vi "ArmFeedForward_Example.vi"() -> ()   [LabVIEW 2019]
uses:
  <vilib>/Rock Robotics/WPI/ThirdParty/JAS_Junk/TrajLib/ProfiledPIDController_SetPID.vi
  <vilib>/Rock Robotics/WPI/ThirdParty/JAS_Junk/TrajLib/ProfiledPIDController_SetIntegratorRange.vi
  <vilib>/Rock Robotics/WPI/ThirdParty/JAS_Junk/TrajLib/ProfiledPIDController_SetTolerance_PosVel.vi
  <vilib>/Rock Robotics/WPI/ThirdParty/JAS_Junk/TrajLib/ProfiledPIDController_DisableContInput.vi
  <vilib>/Rock Robotics/WPI/ThirdParty/JAS_Junk/TrajLib/ProfiledPIDController_EnableContInput.vi
  <vilib>/Rock Robotics/WPI/ThirdParty/JAS_Junk/TrajLib/ProfiledPIDController_Reset_PosOnly.vi
  <vilib>/Rock Robotics/WPI/ThirdParty/JAS_Junk/TrajLib/ProfiledPIDController_NewPeriod.vi
  <vilib>/Rock Robotics/WPI/ThirdParty/JAS_Junk/TrajLib/ProfiledPIDController_Calculate_Meas_Goal.vi
  <vilib>/Rock Robotics/WPI/ThirdParty/JAS_Junk/TrajLib/ProfiledPIDController_AtGoal.vi
  <vilib>/Rock Robotics/WPI/ThirdParty/JAS_Junk/TrajLib/ProfiledPIDController_AtSetpoint.vi
  <vilib>/Rock Robotics/WPI/ThirdParty/JAS_Junk/TrajLib/ProfiledPIDController_SetConstraints.vi
  <vilib>/Rock Robotics/WPI/ThirdParty/JAS_Junk/TrajLib/PIDController_SetPID.vi
  <vilib>/Rock Robotics/WPI/ThirdParty/JAS_Junk/TrajLib/PIDController_SetIntegratorRange.vi
  <vilib>/Rock Robotics/WPI/ThirdParty/JAS_Junk/TrajLib/PIDController_SetTolerancePandV.vi
  <vilib>/Rock Robotics/WPI/ThirdParty/JAS_Junk/TrajLib/PIDController_DisableContinousInput.vi
  <vilib>/Rock Robotics/WPI/ThirdParty/JAS_Junk/TrajLib/PIDController_EnableContinousInput.vi
  <vilib>/Rock Robotics/WPI/ThirdParty/JAS_Junk/TrajLib/TrapProfState_New.vi
  <vilib>/Rock Robotics/WPI/ThirdParty/JAS_Junk/TrajLib/ProfiledPIDController_Reset.vi
  <vilib>/Rock Robotics/WPI/ThirdParty/JAS_Junk/TrajLib/PIDController_NewPeriod.vi
  <vilib>/Rock Robotics/SystemInterfaces/NetworkCommunication/NetComm_UsageReport_report.vi
  <vilib>/Rock Robotics/WPI/ThirdParty/JAS_Junk/TrajLib/ProfiledPIDController_SetGoal_PosOnly.vi
  <vilib>/Rock Robotics/WPI/ThirdParty/JAS_Junk/TrajLib/ProfiledPIDController_Calculate_Meas.vi
  <vilib>/Rock Robotics/WPI/ThirdParty/JAS_Junk/TrajLib/TrapProfState_Equals.vi
  <vilib>/Rock Robotics/WPI/ThirdParty/JAS_Junk/TrajLib/PIDController_AtSetpoint.vi
  <vilib>/Rock Robotics/WPI/ThirdParty/JAS_Junk/TrajLib/PIDController_Reset.vi
  <vilib>/Rock Robotics/WPI/ThirdParty/JAS_Junk/TrajLib/ProfiledPIDController_SetGoal.vi
  <vilib>/Rock Robotics/WPI/ThirdParty/JAS_Junk/TrajLib/PIDController_Calculate_SP_PV.vi
  <vilib>/Rock Robotics/WPI/ThirdParty/JAS_Junk/TrajLib/TrapProfile_New.vi
  <vilib>/Rock Robotics/WPI/ThirdParty/JAS_Junk/TrajLib/ProfiledPIDController_GetPeriod.vi
  <vilib>/Rock Robotics/WPI/ThirdParty/JAS_Junk/TrajLib/TrapProfile_Calculate.vi
  <vilib>/Rock Robotics/WPI/ThirdParty/JAS_Junk/TrajLib/ControllerUtil_GetModulusError.vi
  <vilib>/Rock Robotics/WPI/ThirdParty/JAS_Junk/TrajLib/PIDController_SetSetpoint.vi
  <vilib>/Rock Robotics/WPI/ThirdParty/JAS_Junk/TrajLib/PIDController_Calculate_PV.vi
  <vilib>/Rock Robotics/WPI/ThirdParty/JAS_Junk/TrajLib/TrapProfile_ShouldFlipAcceleration.vi
  <vilib>/Rock Robotics/WPI/ThirdParty/JAS_Junk/TrajLib/TrapProfile_Direct.vi
  <vilib>/Rock Robotics/WPI/ThirdParty/JAS_Junk/TrajLib/PIDController_GetPeriod.vi
  <vilib>/Rock Robotics/WPI/ThirdParty/JAS_Junk/TrajLib/Util_LibraryGlobals.vi
  <vilib>/Rock Robotics/WPI/ThirdParty/JAS_Junk/TrajLib/Trajectory_Library.lvlib
panel:
  in  "Tab Control":T1(tab)
  in  "Arm Posistion\nDemand SP\nRadians":dbl(slide) scale=-1.0..4.0
  out "Battery Voltage":dbl format="%20.3f"
  out "CO Chart":cluster{dbl, "Voltage":dbl}(graph)
  out "Arm Position\nMeasured PV\nRadians":dbl(slide) scale=-1.0..4.0
  out "Arm Angle\nRad":dbl format="%20.3f"
  out "Arm Velocity\nRad/Sec":dbl format="%20.3f"
  out "PV Chart":T2(graph)
  out "Motor Dmd (CO)":dbl format="%20.3f"
  out "At Top":bool
  out "At Bottom":bool
  out "Motor Amps":dbl format="%20.3f"
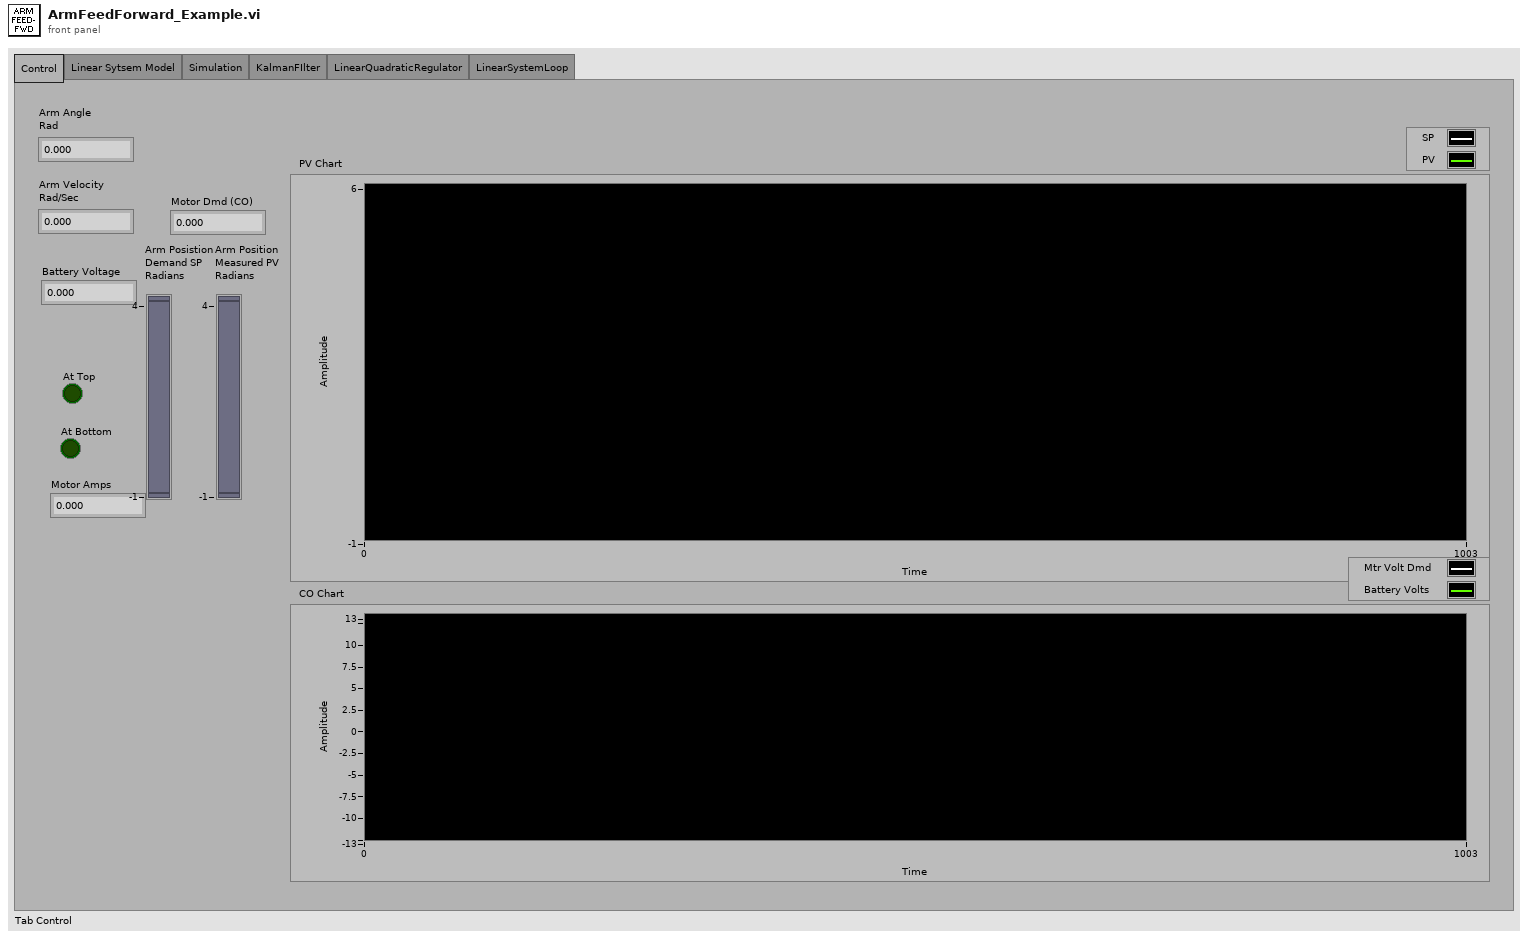
[diagram p1: front panel]
types:
  T1 = enum32{"Control", "Linear Sytsem Model", "Simulation", "KalmanFIlter", "LinearQuadraticRegulator", "LinearSystemLoop"}
  T2 = cluster{"Arm Posistion\nDemand SP\nRadians":dbl, "ArmAngle_Rad":dbl}
  T3 = typedef "Trajectory_Library.lvlib/SINGLE_JOINT_ARM_SIM.ctl" = cluster{"Arm_LinearSystem":T4, "GearBox":T7, "Gearing":dbl, "R_ArmLength_M":dbl, "MinAngle_Rad":dbl, "MaxAngle_Rad":dbl, "ArmMass_Kg":dbl, "SimulateGravity":bool}
  T4 = typedef "Trajectory_Library.lvlib/LINEAR_SYSTEM_SIM.ctl" = cluster{"m_Plant":T5, "m_X":T6, "m_Y":T6, "m_U":T6, "MeasureStdDev":T6}
  T5 = typedef "Trajectory_Library.lvlib/LINEAR_SYSTEM.ctl" = cluster{"m_A":T6, "m_B":T6, "m_C":T6, "m_D":T6, "States":i32, "Inputs":i32, "Outputs":i32}
  T6 = typedef "NI_Matrix.lvlib/RealMatrix.ctl" = dbl[][]
  T7 = typedef "Trajectory_Library.lvlib/DCMOTOR.CTL" = cluster{"nominalVoltage_Volts":dbl, "StallTorque_NM":dbl, "StallCurrent_Amps":dbl, "FreeCurrent_Amps":dbl, "FreeSpeed_RadPerSec":dbl, "R_Ohms":dbl, "KvINV_RadPerSecPerVolt":dbl, "Kt_NMPerAmp":dbl, "L_H":dbl, "Jr_KgM2":dbl}
  T8 = typedef "Trajectory_Library.lvlib/ARM_FF.ctl" = cluster{"Ks":dbl, "Kv":dbl, "Ka":dbl, "kCos":dbl}
  T9 = typedef "Trajectory_Library.lvlib/PID_TUNING.ctl" = cluster{"Kp":dbl, "Ki":dbl, "Kd":dbl, "MaximumIntegral":dbl, "MinimumIntegral":dbl}
  T10 = typedef "Trajectory_Library.lvlib/PID_INPUT_LIMITS.ctl" = cluster{"MaxInput":dbl, "MinInput":dbl, "Continuous":bool}
  T11 = typedef "Trajectory_Library.lvlib/TRAPEZOID_PROFILE_CONSTRAINT.ctl" = cluster{"MaxVelocity":dbl, "MaxAcceleration":dbl}
  T12 = cluster{"CO-ControlOutput":dbl, "Actual Battery Voltage":dbl}
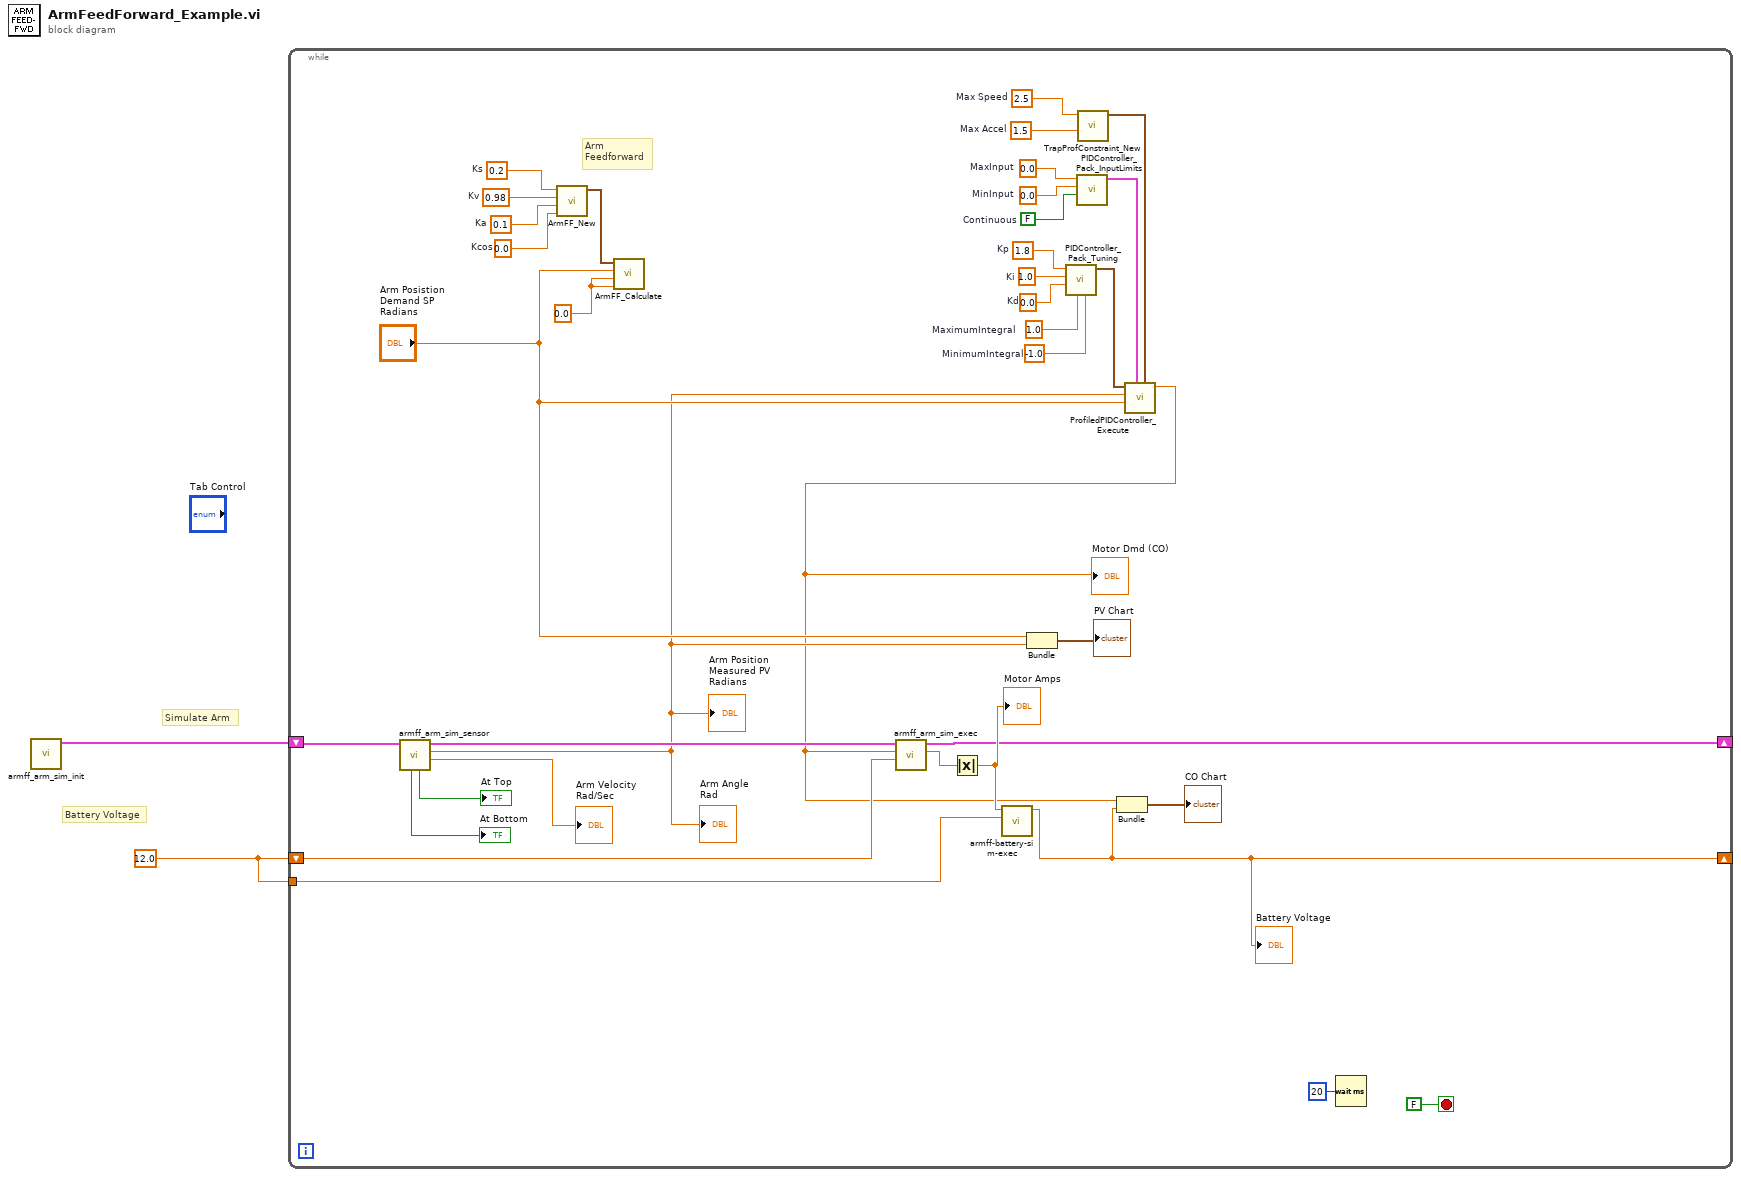
[diagram p0: block diagram]
diagram:
  w2 = 12.0
  # "Simulate Arm"
  # "Battery Voltage"
  n1 = call "armff_arm_sim_init.vi"() -> ("SingleJointArmSim"=w1:T3)  [unwired: 11 in]
  n2 = while {
    shift-right: [w26] -> _
    shift-left: w1 -> [w25]
    shift-right: [w35] -> _
    shift-left: w2 -> [w19]
    tunnel: w2 -> [w32]
    stop <- FALSE stop-if-true
    w18 = 2.5  # Max Speed
    w17 = 1.5  # Max Accel
    w15 = 0.0  # MaxInput
    w14 = 0.0  # MinInput
    w13 = FALSE  # Continuous
    w12 = 1.8  # Kp
    w11 = 1.0  # Ki
    w10 = 0.0  # Kd
    w9 = 1.0  # MaximumIntegral
    w8 = -1.0  # MinimumIntegral
    w24 = 0.0 ("VelocityRadiansPerSec")
    w30 = 0.2  # Ks
    w29 = 0.98  # Kv
    w28 = 0.1  # Ka
    w27 = 0.0  # Kcos
    # "Arm\nFeedforward"
    n3 = call "armff_arm_sim_sensor.vi"("SingleJointArmSim"=w25) -> ("Velocity_RadsPerSec"=→"Arm Velocity\nRad/Sec":dbl, "ArmAngle_Rad"=w4:dbl, "out Arm Sim"=w20:T3, "At HIgh LImit"=→"At Top":bool, "AtLowLimit"=→"At Bottom":bool)  [unwired: 6 in]
    "Arm Position\nMeasured PV\nRadians" <- w4
    "Arm Angle\nRad" <- w4
    n4 = call <vilib>:"ArmFF_New.vi"("Kcos"=w27, "Ka"=w28, "Kv"=w29, "Ks"=w30) -> ("ARM_FF"=w31:T8)  [unwired: 7 in]
    n5 = call <vilib>:"ArmFF_Calculate.vi"("AccelRadPerSecSquared"=w24, "VelocityRadiansPerSec"=w24, "PositionRadians"="Arm Posistion\nDemand SP\nRadians", "in ARM_FF"=w31) -> ()  [unwired: 7 in, 1 out]
    n6 = Bundle("Arm Posistion\nDemand SP\nRadians"="Arm Posistion\nDemand SP\nRadians", "ArmAngle_Rad"=w4) -> (→"PV Chart":T2)  [unwired: 1 in]
    n7 = call <vilib>:"PIDController_Pack_Tuning.vi"("MinimumIntegral"=w8, "MaximumIntegral"=w9, "Kd"=w10, "Ki"=w11, "Kp"=w12) -> ("PID Tuning"=w7:T9)  [unwired: 6 in]
    n8 = call <vilib>:"PIDController_Pack_InputLimits.vi"("Continuous"=w13, "MinInput"=w14, "MaxInput"=w15) -> ("PID Input Limits"=w6:T10)  [unwired: 8 in]
    n9 = call <vilib>:"TrapProfConstraint_New.vi"("Max Accel"=w17, "Max Speed (M/S)"=w18) -> ("TRAPEZOID_PROFILE_CONSTRAINT"=w16:T11)  [unwired: 9 in]
    n10 = call <vilib>:"ProfiledPIDController_Execute.vi"("Constraints"=w16, "PID Input Limits"=w6, "SP-SetPoint Goal"="Arm Posistion\nDemand SP\nRadians", "PV-Measurement"=w4, "PID Tuning"=w7) -> ("CO-ControlOutput"=w3:dbl)  [unwired: 3 in, 3 out]
    "Motor Dmd (CO)" <- w3
    n11 = call "armff_arm_sim_exec.vi"("Current Battery Volltage"=w19, "Motor Dmd SP"=w3, "out Arm Sim"=w20) -> ("Current_Amps"=w34:dbl, "out SingleJointArmSim"=w26:T3)  [unwired: 7 in]
    n12 = Absolute Value(x=w34) -> (abs(x)=w33:dbl)
    "Motor Amps" <- w33
    n13 = call "armff-battery-sim-exec.vi"("Nominal Battery Voltge"=w32, "Current"=w33) -> ("Actual Battery Voltage"=w35:dbl)  [unwired: 9 in]
    "Battery Voltage" <- w35
    n14 = Bundle("CO-ControlOutput"=w3, "Actual Battery Voltage"=w35) -> (→"CO Chart":T12)  [unwired: 1 in]
    n15 = Wait (ms)(milliseconds to wait=u32 20) -> ()  [unwired: 1 out]
  }
